vi "Decimation.vi"(11 "Decimation Factor":i32) -> (3 "Trigger":bool)   [LabVIEW 2011]
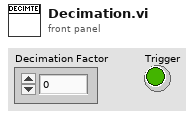
[diagram p1: front panel]
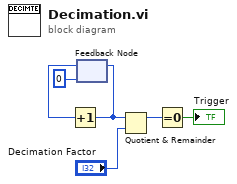
[diagram p0: block diagram]
diagram:
  n1 = feedback #1(0) -> (w5:i32)
  n2 = Increment(x=w5) -> (x+1=w4:i32)
  n3 = feedback-in #1(w4) -> ()
  n4 = Quotient & Remainder(x=w4, y="Decimation Factor") -> (x-y*floor(x/y)=w1:i32)  [unwired: 1 out]
  n5 = Equal To 0?(x=w1) -> (x = 0?=→"Trigger":bool)
